vi "_SILAR 2016.vi"() -> ()   [LabVIEW 2016]
uses:
  <vilib>/LabVIEW Interface for Arduino/LabVIEW Interface for Arduino.lvlib
panel:
  in  "?":T1(tab)
  in  "Запись в файл":bool=TRUE
  in  "Необходимая температура":dbl[](array[numeric])=[90.0, 0.0, 0.0, 0.0]
  in  "Кол-во погружений в каждый стакан":i32[](array[numeric])=[1, 1, 1, 1]
  in  "Кол-во жидкости в каждом стакане [мл]":dbl[](array[numeric])=[70.0, 70.0, 70.0, 70.0]
  in  "Глубина погружения в раствор [мм]":dbl[](array[numeric])=[5.0, 5.0, 5.0, 5.0]
  in  "Опускания подложки до раствора":dbl[](array[numeric])=[2.9, 2.9, 2.9, 2.9]
  in  "Опускания подложки в растворе":dbl[](array[numeric])=[2.9, 2.9, 2.9, 2.9]
  in  "Подъема подложки из раствора":dbl[](array[numeric])=[2.9, 2.9, 2.9, 2.9]
  in  "Подъема подложки над раствором":dbl[](array[numeric])=[2.9, 2.9, 2.9, 2.9]
  in  "Нахождения в растворе":dbl[](array[numeric])=[1.0, 1.0, 1.0, 1.0] caption="Время нахождения в растворе (секунды)"
  in  "Задержки после подъема из раствора":dbl[](array[numeric])=[0.0, 0.0, 0.0, 0.0]
  in  "Оператор":string="Матюшкин"
  in  "Образец":string
  in  "COM порт":refnum<visa-resource-name>="COM6"
  in  "Кол-во циклов наслаивания":i32=1
  in  "Кол-во используемых растворов":i32(ring)=1 items=["Один"=1, "Два"=2, "Три"=3, "Четыре"=4]
  in  "Высота стакана [мм]":dbl=81.2
  in  "Высота подложки [мм]":dbl=22.0
  in  "Режим погружения подложки":u16(ring) items=["Частичный", "Полный"]
  in  "Запуск":bool
  in  "Выход из программы":bool
  in  "Включение нагрева":bool=TRUE
  in  "Считать данные":bool
  in  "Путь к файлу":path=path "C:/Users/user/Dropbox/SILAR/Devic"
  out "Время Темп":dbl=7.964
  out "Текущая темп. 3":dbl
  out "Нагрева":timestamp=timestamp(-14399.531 s since 1904-01-01) format="%<%H:%M:%S>T"
  out "До конца процесса":timestamp=timestamp(-14399.531 s since 1904-01-01) format="%<%H:%M:%S>T"
  out "С начала процесса":timestamp=timestamp(-14399.531 s since 1904-01-01) format="%<%H:%M:%S>T"
  out "Всего процесса":timestamp=timestamp(-14399.531 s since 1904-01-01) format="%<%H:%M:%S>T"
  out "Процесс выполнения":dbl(slide) scale=0.0..1.0
  out "Текущая темп. 1":dbl
  out "Текущая темп. 4":dbl
  out "Текущая темп. 2":dbl
  out "Текущий цикл":dbl
  out "Всего циклов":i32=2
  in  "Запуск процесса":bool
  out "Indic":bool[](array[boolean])
  out "2":bool
  out "1":bool
  out "3":bool
  out "Стакакан 1":dbl(slide) scale=0.0..81.0
  out "Термометр 1":dbl(slide) scale=20.0..90.0 scale format="%#_3g"
  out "Стакакан 2":dbl(slide) scale=0.0..81.0
  out "Термометр 2":dbl(slide) scale=20.0..90.0 scale format="%#_3g"
  out "Стакакан 3":dbl(slide) scale=0.0..81.0
  out "Термометр 3":dbl(slide) scale=20.0..90.0 scale format="%#_3g"
  out "Стакакан 4":dbl(slide) scale=0.0..81.0
  out "Термометр 4":dbl(slide) scale=20.0..90.0 scale format="%#_3g"
  out "Текущее кол-во погружений в каждый стакан":i32[](array[numeric])
  in  "Остановка":bool
  out "Нагрев завершен":bool
  out "Нагрев включен":bool
  # "Вкл"
  # "Выкл"
  # "Параметры на каждом стакане"
  # "1              2             3             4"
  # "Температура [градусы Цельсия]"
  # "Скорость [мм/с] (max 2,9 мм/с)"
  # "Время [c]"
  # "Параметры процесса"
  # "Вкл"
  # "Выкл"
  # "Считывание параметров процесса"
  # "Время"
  # "1"
  # "2"
  # "3"
  # "4"
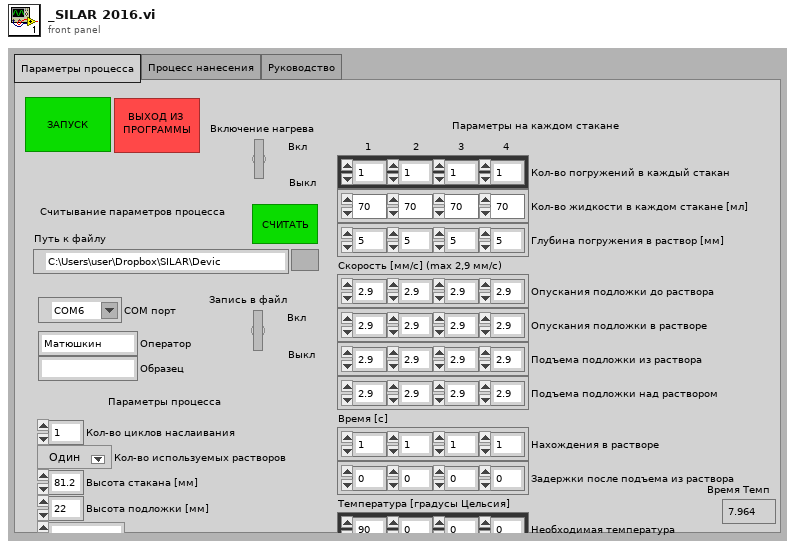
[diagram p1: front panel]
types:
  T1 = enum32{"Параметры процесса", "Процесс нанесения", "Руководство"}
  T2 = typedef "LabVIEW Interface for Arduino.lvlib/Arduino Resource.ctl" = cluster{"VISA resource":refnum<visa-resource-name>, "Board Type":T3, "Connection Type":enum8{"USB / Serial"}, "Bytes Per Packet (15)":u8}
  T3 = typedef "LabVIEW Interface for Arduino.lvlib/Board Type.ctl" = enum16{"Uno", "Dimuelanove w/Atmega 328", "Mega 2560"}
  T4 = enum32{"Параметры процесса", "Процесс нанесения"}
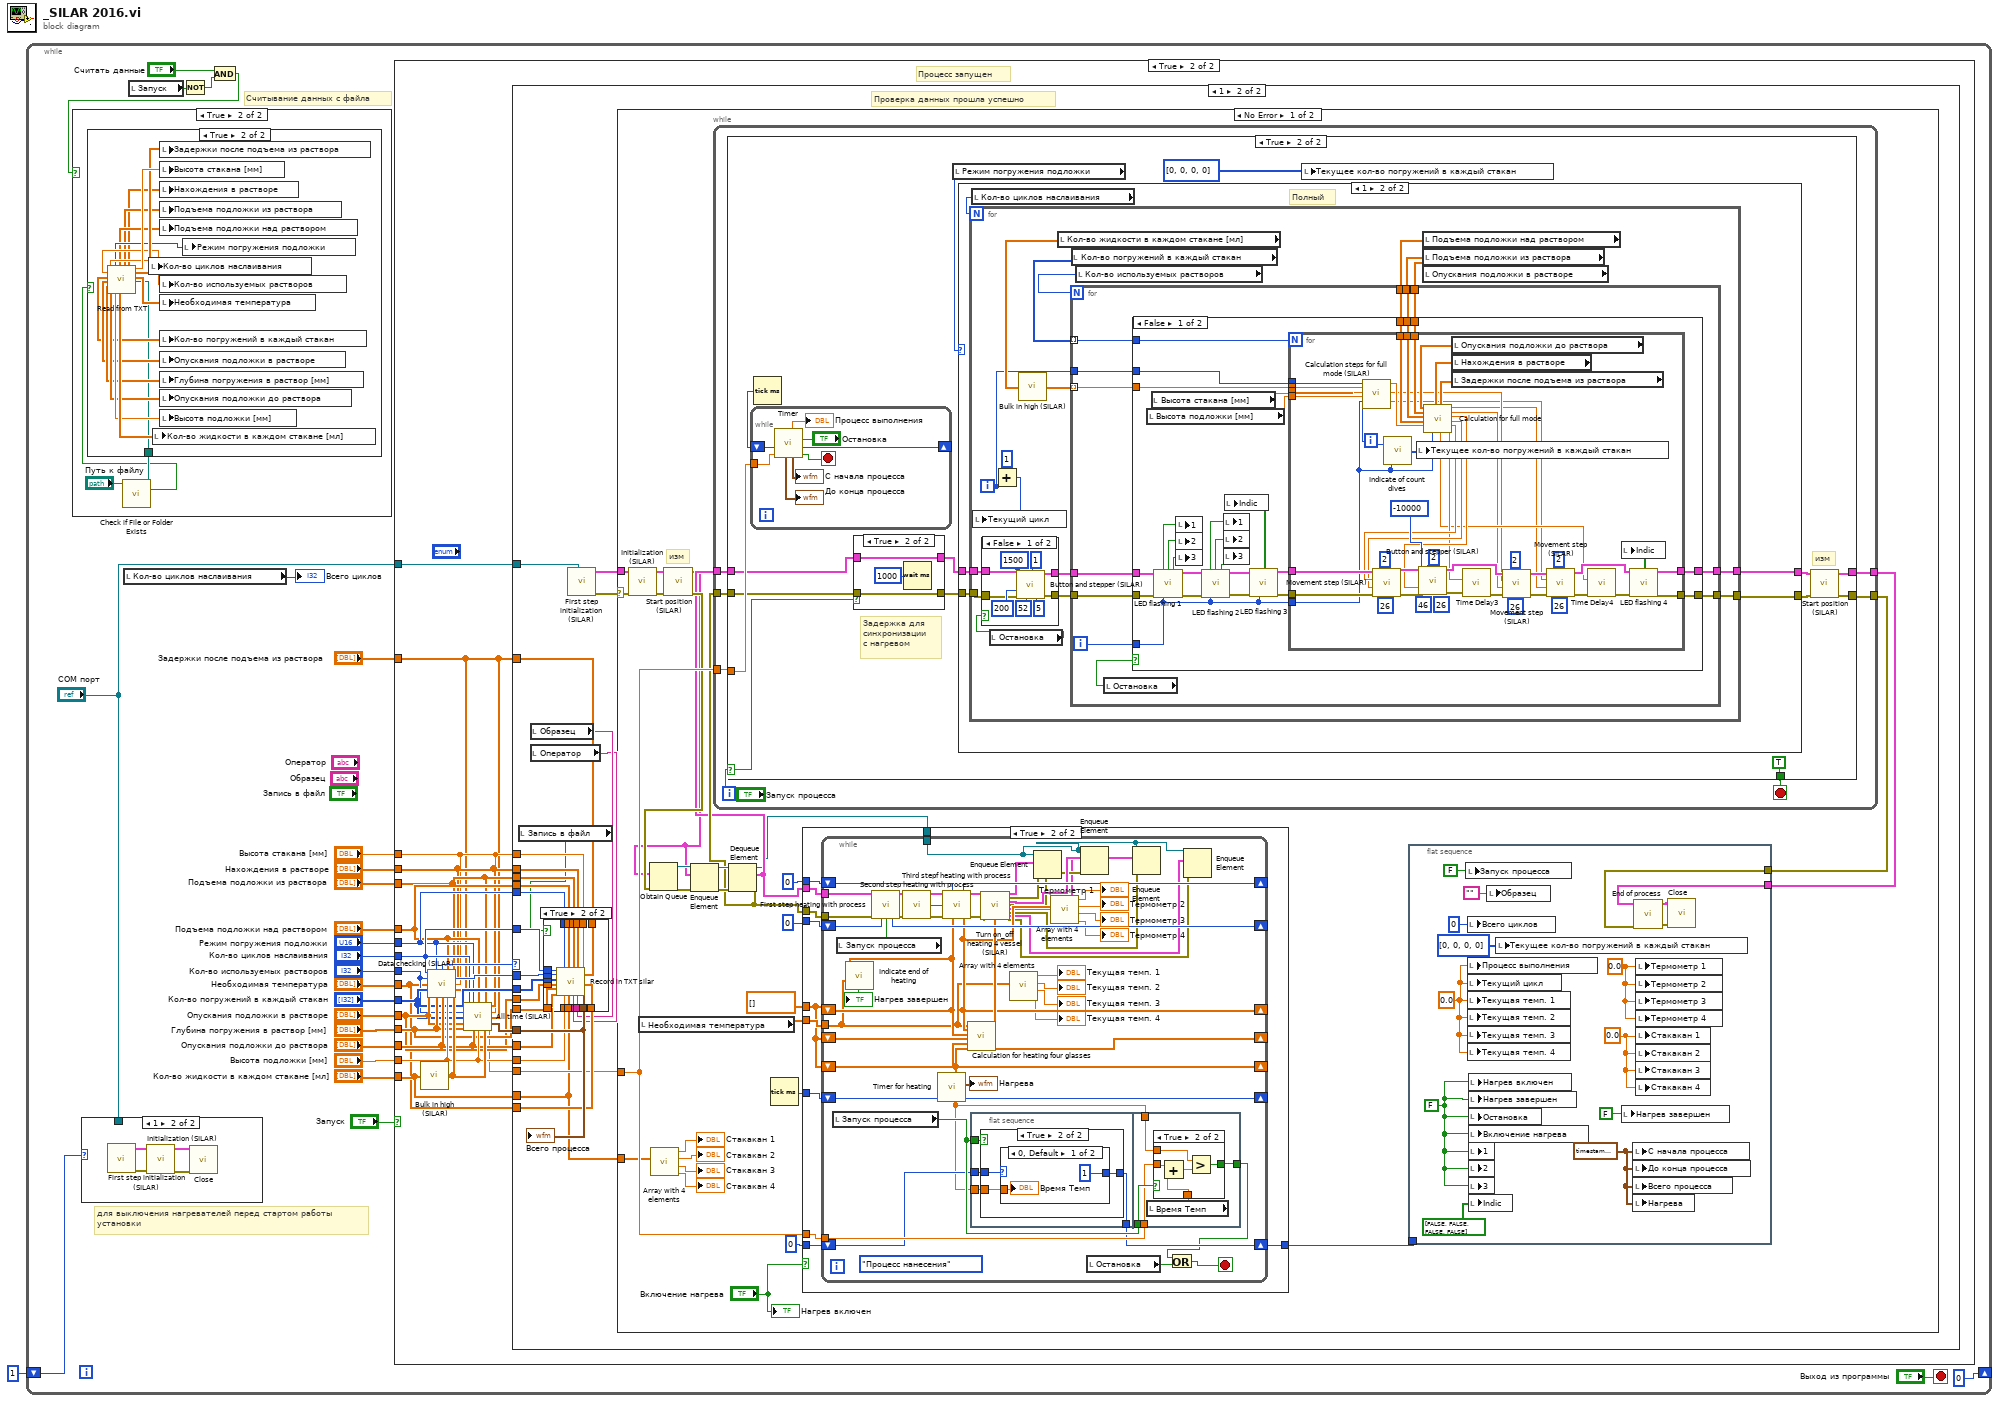
[diagram p0: block diagram]
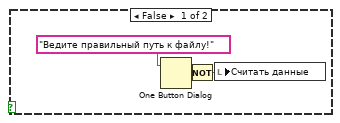
[diagram p4: hidden frame]
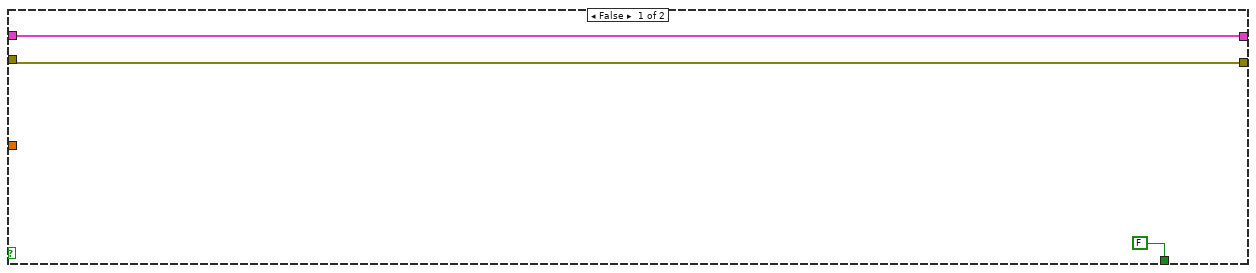
[diagram p8: hidden frame]
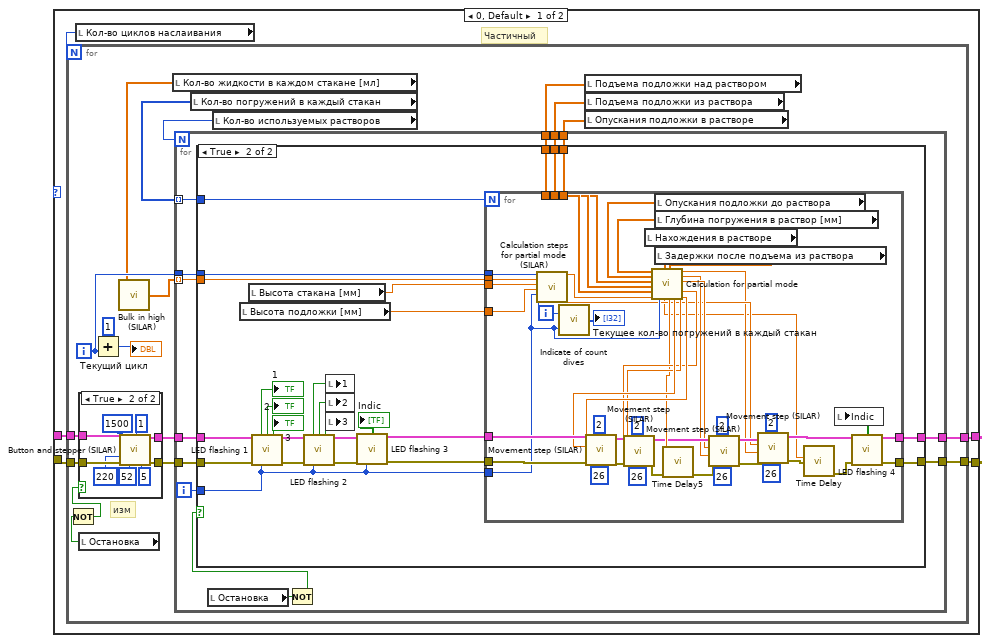
[diagram p10: hidden frame]
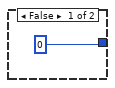
[diagram p15: hidden frame]
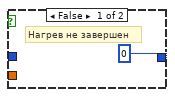
[diagram p16: hidden frame]
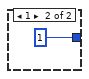
[diagram p17: hidden frame]
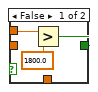
[diagram p18: hidden frame]
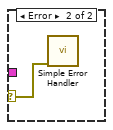
[diagram p19: hidden frame]
diagram:
  n1 = while {
    shift-right: [0 ("Всего циклов")] -> _
    shift-left: 1 -> [w3]
    stop <- "Выход из программы" stop-if-true
    # "для выключения нагревателей перед стартом работы\nустановки"
    # "Cчитывание данных с файла"
    n2 = case shown="1" w3 {
      tunnel: "COM порт" -> [_ _]
      frame 0, Default {
      }
      frame 1 {
        n3 = call "First step initialization (SILAR).vi"() -> ("Error Out"=w29:errorcluster, "Arduino Resource Out"=w30:T2)  [unwired: 10 in]
        n4 = call "Initialization (SILAR).vi"("Error In"=w29, "Arduino Resource In"=w30) -> ("Error Out"=w27:errorcluster, "Arduino Resource Out"=w28:T2)  [unwired: 8 in]
        n5 = call <vilib>:"Close.vi"("Arduino Resource"=w28, "error in"=w27) -> ()  [unwired: 13 in, 1 out]
      }
    }
    n6 = local read "Кол-во циклов наслаивания"() -> (→"Всего циклов":i32)
    n7 = local read "Запуск"() -> (w25:bool)
    n8 = Not(x=w25) -> (.not. x?=w22:bool)
    n9 = And(x="Считать данные", y=w22) -> (x .and. y?=w24:bool)
    n10 = case shown="True" w24 {
      frame False {
      }
      frame True {
        n11 = call <vilib>:"Check if File or Folder Exists.vi"("path"="Путь к файлу") -> ("file or folder exists?"=w31:bool, "dup path"=w32:path)  [unwired: 8 in, 1 out]
        n12 = case shown="True" w31 {
          tunnel: w32 -> [_ w37]
          frame False {
            n13 = One Button Dialog(message="Ведите правильный путь к файлу!") -> (true=w34:bool)  [unwired: 1 in]
            n14 = Not(x=w34) -> (.not. x?=w35:bool)
            n15 = local write "Считать данные"(w35) -> ()
          }
          frame True {
            n16 = call "Read from TXT.vi"("Файл с параметрами"=w37) -> ("Кол-во циклов наслаивания"=w42:dbl, "Кол-во используемых растворов"=w43:dbl, "Кол-во погружений в каждый раствор:"=w44:dbl[], "Опускания подложки в растворе:"=w45:dbl[], "Глубина погружения в раствор [мм]:"=w46:dbl[], "Опускания подложки до раствора:"=w47:dbl[], "Режим погружения"=w41:i32, "Высота подложки [мм]"=w48:dbl, "Подъем подложки над раствором:"=w40:dbl[], "Кол-во жидкости в стакане [мл]:"=w49:dbl[], "Подъема подложки из раствора:"=w39:dbl[], "Нахождения в растворе:"=w38:dbl[], "Высота стакана [мм]"=w52:dbl, "Задержки после подъема из раствора:"=w51:dbl[], "Температура в стаканах:"=w50:dbl[])  [unwired: 3 in, 1 out]
            n17 = local write "Кол-во циклов наслаивания"(w42) -> ()
            n18 = local write "Кол-во жидкости в каждом стакане [мл]"(w49) -> ()
            n19 = local write "Задержки после подъема из раствора"(w51) -> ()
            n20 = local write "Высота стакана [мм]"(w52) -> ()
            n21 = local write "Нахождения в растворе"(w38) -> ()
            n22 = local write "Подъема подложки из раствора"(w39) -> ()
            n23 = local write "Подъема подложки над раствором"(w40) -> ()
            n24 = local write "Кол-во используемых растворов"(w43) -> ()
            n25 = local write "Необходимая температура"(w50) -> ()
            n26 = local write "Кол-во погружений в каждый стакан"(w44) -> ()
            n27 = local write "Опускания подложки в растворе"(w45) -> ()
            n28 = local write "Глубина погружения в раствор [мм]"(w46) -> ()
            n29 = local write "Опускания подложки до раствора"(w47) -> ()
            n30 = local write "Высота подложки [мм]"(w48) -> ()
            n31 = local write "Режим погружения подложки"(w41) -> ()
          }
        }
      }
    }
    n32 = case shown="True" "Запуск" {
      tunnel: "Задержки после подъема из раствора" -> [_ w56]
      tunnel: "Высота стакана [мм]" -> [_ w57]
      tunnel: "Нахождения в растворе" -> [_ w58]
      tunnel: "Подъема подложки из раствора" -> [_ w59]
      tunnel: "Подъема подложки над раствором" -> [_ w60]
      tunnel: "Режим погружения подложки" -> [_ w61]
      tunnel: "Кол-во циклов наслаивания" -> [_ w62]
      tunnel: "Кол-во используемых растворов" -> [_ w63]
      tunnel: "Необходимая температура" -> [_ w55]
      tunnel: "Кол-во погружений в каждый стакан" -> [_ w64]
      tunnel: "Опускания подложки в растворе" -> [_ w65]
      tunnel: "Глубина погружения в раствор [мм]" -> [_ w66]
      tunnel: "Опускания подложки до раствора" -> [_ w67]
      tunnel: "Высота подложки [мм]" -> [_ w68]
      tunnel: "Кол-во жидкости в каждом стакане [мл]" -> [_ w69]
      tunnel: "COM порт" -> [_ w53]
      frame False {
      }
      frame True {
        # "Процесс запущен"
        n33 = call "Bulk in high (SILAR).vi"("Кол-во жидкости в каждом стакане (мл)"=w69) -> ("Кол-во жидкости в каждом стакане (мм)"=w72:dbl[])
        n34 = call "Data checking (SILAR).vi"("Необходимое кол-во циклов"=w62, "Режим погружения подложки"=w61, "Подъема подложки над раствором"=w60, "Подъема подложки из раствора"=w59, "Кол-во используемых растворов"=w63, "Время нахождения в растворе (секунды)"=w58, "Необходимая температура"=w55, "Высота стакана"=w57, "Кол-во погружений в каждый стакан за один цикл"=w64, "Задержки после подъема из раствора"=w56, "Опускания подложки в раствор"=w65, "Глубина погружения в раствор"=w66, "Опускания подложки до раствора"=w67, "Высота подложки"=w68, "Кол-во жидкости в каждом стакане (мм)"=w72) -> ("ПРОВЕРКА"=w71:i16)
        n35 = call "All time (SILAR).vi"("Необходимое кол-во циклов"=w62, "Режим погружения подложки"=w61, "Подъема подложки над раствором"=w60, "Подъема подложки из раствора"=w59, "Нахождения в растворе (секунды)"=w58, "Кол-во используемых растворов"=w63, "Высота стакана (мм)"=w57, "Кол-во погружений в каждый стакан за один цикл"=w64, "Задержка после подъема из раствора (секунды)"=w56, "Опускания подложки в раствор"=w65, "Глубина погружения в раствор (мм)"=w66, "Опускания подложки до раствора"=w67, "Высота подложки (мм)"=w68, "Кол-во жидкости в каждом стакане (мм)"=w72) -> (10:"Все время"=w70:timestamp, 15:"Все время"=w54:dbl)
        n36 = case shown="1" w71 {
          tunnel: w70 -> [_ w95]
          tunnel: w69 -> [_ w77]
          tunnel: w68 -> [_ w94]
          tunnel: w67 -> [_ w93]
          tunnel: w66 -> [_ w92]
          tunnel: w65 -> [_ w91]
          tunnel: w64 -> [_ w90]
          tunnel: w63 -> [_ w89]
          tunnel: w62 -> [_ w88]
          tunnel: w61 -> [_ w87]
          tunnel: w60 -> [_ w86]
          tunnel: w59 -> [_ w85]
          tunnel: w58 -> [_ w84]
          tunnel: w57 -> [_ w83]
          tunnel: w56 -> [_ w82]
          tunnel: w55 -> [_ w81]
          tunnel: w54 -> [_ w78]
          tunnel: w53 -> [_ w76]
          frame 0, Default {
          }
          frame 1 {
            # "Проверка данных прошла успешно"
            n37 = local read "Запись в файл"() -> (w75:bool)
            n38 = local read "Образец"() -> (w74:string)
            n39 = local read "Оператор"() -> (w73:string)
            n40 = case shown="True" w75 {
              tunnel: w73 -> [_ w113]
              tunnel: w74 -> [_ w112]
              tunnel: w95 -> [_ w111]
              tunnel: w94 -> [_ w110]
              tunnel: w93 -> [_ w109]
              tunnel: w92 -> [_ w108]
              tunnel: w91 -> [_ w107]
              tunnel: w90 -> [_ w106]
              tunnel: w89 -> [_ w105]
              tunnel: w88 -> [_ w104]
              tunnel: w87 -> [_ w103]
              tunnel: w86 -> [_ w102]
              tunnel: w85 -> [_ w101]
              tunnel: w84 -> [_ w100]
              tunnel: w83 -> [_ w99]
              tunnel: w82 -> [_ w98]
              tunnel: w81 -> [_ w97]
              tunnel: w77 -> [_ w96]
              frame False {
              }
              frame True {
                n41 = call "Record in TXT silar.vi"("Кол-во циклов"=w104, "Кол-во используемых растворов"=w105, "Кол-во погружений в каждый стакан"=w106, "Опускания подложки в растворе"=w107, "Глубина погружения в раствор [мм]"=w108, "Опускания подложки до раствора"=w109, "Режим погружения подложки"=w103, "Высота подложки [мм]"=w110, "Подъема подложки над раствором"=w102, "Кол-во жидкости в каждом стакане [мл]"=w96, "Подъема подложки из раствора"=w101, "Оператор"=w113, "Нахождения в растворе"=w100, "Получаемый образец"=w112, "Высота стакана [мм]"=w99, "Задержки после подъема из раствора"=w98, "Необходимая температура"=w97, "Все время процесса"=w111) -> ()  [unwired: 2 in]
              }
            }
            n42 = call "First step initialization (SILAR).vi"("COM порт"=w76) -> ("Error Out"=w80:errorcluster, "Arduino Resource Out"=w79:T2)  [unwired: 9 in]
            n43 = case shown="No Error" w80 {
              selector: w80 -> [w141 w524]
              tunnel: w79 -> [w142 _]
              tunnel: w78 -> [w132 _]
              tunnel: w77 -> [w131 _]
              frame No Error {
                # "изм"
                n44 = call "Initialization (SILAR).vi"("Error In"=w141, "Arduino Resource In"=w142) -> ("Error Out"=w139:errorcluster, "Arduino Resource Out"=w140:T2)  [unwired: 8 in]
                n45 = local read "Необходимая температура"() -> (w138:dbl[])
                n46 = call "Array with 4 elements.vi"("Array with 4 elements"=w131) -> ("element 3"=→"Стакакан 4":dbl, "element 2"=→"Стакакан 3":dbl, "element 1"=→"Стакакан 2":dbl, "element 0"=→"Стакакан 1":dbl)  [unwired: 7 in]
                n47 = call "Start position (SILAR).vi"("Error In"=w139, "Arduino Resource In"=w140) -> ("Error Out"=w119:errorcluster, "Arduino Resource Out"=w115:T2)  [unwired: 8 in]
                n48 = Obtain Queue(element data type=w115, error in (no error)=w119) -> (queue out=w123:refnum<queue>, error out=w120:errorcluster)  [unwired: 3 in, 1 out]
                n49 = Enqueue Element(queue=w123, element=w115, error in (no error)=w120) -> (queue out=w122:refnum<queue>, error out=w121:errorcluster)  [unwired: 1 in, 1 out]
                n50 = Dequeue Element(queue=w122, error in (no error)=w121) -> (queue out=w116:refnum<queue>, element=w117:T2, error out=w118:errorcluster)  [unwired: 1 in, 1 out]
                n51 = while {
                  tunnel: w132 -> [w164]
                  tunnel: [w163] -> w129
                  tunnel: [w162] -> w130
                  tunnel: w117 -> [w161]
                  tunnel: w118 -> [w160]
                  stop <- w159 stop-if-true
                  n52 = case shown="True" "Запуск процесса" {
                    selector: "Запуск процесса" -> [_ w172]
                    tunnel: w164 -> [_ w178]
                    tunnel: [w167 w168] -> w163
                    tunnel: [w166 w169] -> w162
                    tunnel: w161 -> [w167 w174]
                    tunnel: w160 -> [w166 w173]
                    tunnel: [FALSE TRUE] -> w159
                    frame False {
                    }
                    frame True {
                      # "изм"
                      # "Задержка для\nсинхронизации\nс нагревом"
                      n53 = Tick Count (ms)() -> (millisecond timer value=w179:u32)
                      n54 = while {
                        shift-right: [w193] -> _
                        shift-left: w179 -> [w194]
                        tunnel: w178 -> [w188]
                        stop <- w192 stop-if-true
                        n55 = call "Timer.vi"("Остановка процесса"="Остановка", "Рассчитанное время"=w188, "shift before"=w194) -> ("end time"=w192:bool, "shift after"=w193:u32, "Время с начала процесса"=→"С начала процесса":timestamp, "Процесс выполнения (шкала)"=→"Процесс выполнения":dbl, "Осталось времени \nдо конца процесса"=→"До конца процесса":timestamp)  [unwired: 4 in]
                      }
                      n56 = case shown="True" w172 {
                        tunnel: [w182 w186] -> w176
                        tunnel: w173 -> [w182 w186]
                        tunnel: w174 -> [w183 w185]
                        tunnel: [w183 w185] -> w175
                        frame False {
                        }
                        frame True {
                          n57 = Wait (ms)(milliseconds to wait=u32 1000) -> ()  [unwired: 1 out]
                        }
                      }
                      n58 = local read "Режим погружения подложки"() -> (w181:u16)
                      n59 = case shown="1" w181 {
                        tunnel: w175 -> [w199 w322]
                        tunnel: w176 -> [w198 w321]
                        tunnel: [w196 w319] -> w171
                        tunnel: [w195 w318] -> w170
                        frame 0, Default {
                          # "Частичный"
                          n60 = local read "Кол-во циклов наслаивания"() -> (w197:i32)
                          n61 = for {
                            N: w197 -> [_]
                            tunnel: w199 -> [w217]
                            tunnel: w198 -> [w216]
                            tunnel: [w203] -> w196
                            tunnel: [w202] -> w195
                            i -> [w209]
                            # "изм"
                            n62 = local read "Остановка"() -> (w200:bool)
                            n63 = Not(x=w200) -> (.not. x?=w201:bool)
                            n64 = case shown="True" w201 {
                              tunnel: w217 -> [w219 w224]
                              tunnel: w216 -> [w218 w223]
                              tunnel: [w218 w222] -> w212
                              tunnel: [w219 w221] -> w211
                              frame False {
                              }
                              frame True {
                                n65 = call "Button and stepper (SILAR).vi"("Arduino Resource In"=w224, "Шаговый двигатель №"=u8 1 ("Stepper #"), "Кол-во шагов"=i16 1500 ("# of Steps to Move"), "Скорость двигателя"=i16 220 ("Set Speed (Steps per Second)"), "Error In"=w223, "Контакт концевика"=u8 52 ("Digital I/O Pin (0)"), "ENABLE контакт"=u8 5 ("ENABLE Pin")) -> ("Arduino Resource Out"=w221:T2, "Error Out"=w222:errorcluster)  [unwired: 7 in]
                              }
                            }
                            n66 = Add(x=1, y=w209) -> (x+y=→"Текущий цикл":i32)
                            n67 = local read "Кол-во жидкости в каждом стакане [мл]"() -> (w208:dbl[])
                            n68 = call "Bulk in high (SILAR).vi"("Кол-во жидкости в каждом стакане (мл)"=w208) -> ("Кол-во жидкости в каждом стакане (мм)"=w207:dbl[])
                            n69 = local read "Кол-во погружений в каждый стакан"() -> (w210:i32[])
                            n70 = local read "Кол-во используемых растворов"() -> (w213:i32)
                            n71 = local read "Подъема подложки над раствором"() -> (w206:dbl[])
                            n72 = local read "Подъема подложки из раствора"() -> (w205:dbl[])
                            n73 = local read "Опускания подложки в растворе"() -> (w204:dbl[])
                            n74 = for {
                              N: w213 -> [_]
                              tunnel: w212 -> [w241]
                              tunnel: w211 -> [w240]
                              tunnel: w210 -> [w239] mode=indexing
                              tunnel: w209 -> [w238]
                              tunnel: w207 -> [w237] mode=indexing
                              tunnel: w206 -> [w236]
                              tunnel: w205 -> [w235]
                              tunnel: w204 -> [w234]
                              tunnel: [w233] -> w203
                              tunnel: [w232] -> w202
                              i -> [w229]
                              n75 = local read "Остановка"() -> (w231:bool)
                              n76 = Not(x=w231) -> (.not. x?=w230:bool)
                              n77 = case shown="True" w230 {
                                tunnel: w241 -> [w242 w269]
                                tunnel: w240 -> [w243 w268]
                                tunnel: w239 -> [_ w267]
                                tunnel: w238 -> [_ w266]
                                tunnel: w237 -> [_ w265]
                                tunnel: w236 -> [_ w260]
                                tunnel: w235 -> [_ w259]
                                tunnel: w234 -> [_ w258]
                                tunnel: [w243 w257] -> w233
                                tunnel: [w242 w256] -> w232
                                tunnel: w229 -> [_ w255]
                                frame False {
                                }
                                frame True {
                                n78 = local read "Высота подложки [мм]"() -> (w263:dbl)
                                n79 = local read "Высота стакана [мм]"() -> (w264:dbl)
                                n80 = call "LED flashing 1.vi"("Arduino Resource In"=w268, "Error Out In"=w269, "Текущий раствор"=w255) -> ("1"=→"1":bool, "2"=→"2":bool, "3"=→"3":bool, "Arduino Resource Out"=w251:T2, "Error Out"=w250:errorcluster)  [unwired: 8 in]
                                n81 = call "LED flashing 2.vi"("Arduino Resource In"=w251, "Error In"=w250, "Текущий раствор"=w255) -> ("1"=w247:bool, "2"=w248:bool, "3"=w249:bool, "Arduino Resource Out"=w246:T2, "Error Out"=w245:errorcluster)  [unwired: 8 in]
                                n82 = local write "1"(w247) -> ()
                                n83 = local write "2"(w248) -> ()
                                n84 = local write "3"(w249) -> ()
                                n85 = call "LED flashing 3.vi"("Arduino Resource In"=w246, "Error In"=w245, "Текущий раствор"=w255) -> ("1           2           3          4"=→"Indic":bool[], "Arduino Resource Out"=w262:T2, "Error Out"=w261:errorcluster)  [unwired: 10 in]
                                n86 = for {
                                N: w267 -> [_]
                                tunnel: w266 -> [w317]
                                tunnel: w265 -> [w316]
                                tunnel: w264 -> [w315]
                                tunnel: w263 -> [w314]
                                tunnel: w255 -> [w309]
                                tunnel: w262 -> [w311]
                                tunnel: w261 -> [w310]
                                tunnel: w260 -> [w307]
                                tunnel: w259 -> [w306]
                                tunnel: w258 -> [w305]
                                tunnel: [w299] -> w257
                                tunnel: [w298] -> w256
                                i -> [w312]
                                n87 = call "Calculation steps for partial mode (SILAR).vi"("Loop iteration для кол-ва циклов"=w317, "Кол-во жидкости в каждом стакане [мм]"=w316, "Высота стакана [мм]"=w315, "Высота подложки [мм]"=w314, "Loop iteration для кол-ва используемых растворов"=w309, "Loop iteration для кол-ва погружений в каждый стакан"=w312) -> ("Кол-во шагов до раствора"=w308:dbl, "Кол-во шагов над раствором"=w283:dbl)  [unwired: 12 in]
                                n88 = call "Indicate of count dives.vi"("Текущий раствор"=w309, "Текущее погружение"=w312) -> ("Текущее кол-во погружений в каждый стакан"=→"Текущее кол-во погружений в каждый стакан":i32[])
                                n89 = local read "Нахождения в растворе"() -> (w302:dbl[])
                                n90 = local read "Опускания подложки до раствора"() -> (w304:dbl[])
                                n91 = local read "Глубина погружения в раствор [мм]"() -> (w303:dbl[])
                                n92 = local read "Задержки после подъема из раствора"() -> (w301:dbl[])
                                n93 = call "Calculation for partial mode.vi"("Глубина погружения в раствор [мм]"=w303, "Опускания подложки до раствора"=w304, "Опускания подложки в растворе"=w305, "Подъема подложки из раствора"=w306, "Подъема подложки над раствором"=w307, "Steps for partial mode"=w308, "Текущий раствор"=w309, "Нахождения в растворе"=w302, "Задержки после подъема из раствора"=w301) -> ("Время задержки после подъема"=w279:dbl, "Время нахождения в растворе"=w290:dbl, "Кол-во шагов 1"=w297:dbl, "Скорость 4"=w282:dbl, "Скорость 3"=w286:dbl, "Кол-во шагов 3"=w287:dbl, "Скорость 2"=w293:dbl, "Кол-во шагов 2"=w292:dbl, "Скорость 1"=w296:dbl)  [unwired: 2 in]
                                n94 = call "Movement step (SILAR).vi"("ENABLE контакт"=u8 26 ("ENABLE Pin"), "Шаговый двигатель №"=u8 2 ("Stepper #"), "Error In"=w310, "Скорость"=w296, "Кол-во шагов"=w297, "Arduino Resource In"=w311) -> ("Error Out"=w294:errorcluster, "Arduino Resource Out"=w295:T2)  [unwired: 4 in]
                                n95 = call "Movement step (SILAR).vi"("ENABLE контакт"=u8 26 ("ENABLE Pin"), "Шаговый двигатель №"=u8 2 ("Stepper #"), "Error In"=w294, "Скорость"=w293, "Кол-во шагов"=w292, "Arduino Resource In"=w295) -> ("Error Out"=w291:errorcluster, "Arduino Resource Out"=w289:T2)  [unwired: 4 in]
                                n96 = call "Time Delay5"("error in (no error)"=w291, "Delay Time (s)"=w290) -> ("error out"=w288:errorcluster)  [unwired: 9 in]
                                n97 = call "Movement step (SILAR).vi"("ENABLE контакт"=u8 26 ("ENABLE Pin"), "Шаговый двигатель №"=u8 2 ("Stepper #"), "Error In"=w288, "Скорость"=w286, "Кол-во шагов"=w287, "Arduino Resource In"=w289) -> ("Error Out"=w284:errorcluster, "Arduino Resource Out"=w285:T2)  [unwired: 4 in]
                                n98 = call "Movement step (SILAR).vi"("ENABLE контакт"=u8 26 ("ENABLE Pin"), "Шаговый двигатель №"=u8 2 ("Stepper #"), "Error In"=w284, "Скорость"=w282, "Кол-во шагов"=w283, "Arduino Resource In"=w285) -> ("Error Out"=w280:errorcluster, "Arduino Resource Out"=w281:T2)  [unwired: 4 in]
                                n99 = call "Time Delay"("error in (no error)"=w280, "Delay Time (s)"=w279) -> ("error out"=w270:errorcluster)  [unwired: 9 in]
                                n100 = call "LED flashing 4.vi"("Arduino Resource In"=w281, "Error In"=w270) -> ("1           2           3          4"=w300:bool[], "Arduino Resource Out"=w299:T2, "Error Out"=w298:errorcluster)  [unwired: 11 in]
                                n101 = local write "Indic"(w300) -> ()
                                }
                                }
                              }
                            }
                          }
                        }
                        frame 1 {
                          # "Полный"
                          n102 = local read "Кол-во циклов наслаивания"() -> (w320:i32)
                          n103 = for {
                            N: w320 -> [_]
                            tunnel: w322 -> [w338]
                            tunnel: w321 -> [w337]
                            tunnel: [w328] -> w319
                            tunnel: [w327] -> w318
                            i -> [w330]
                            n104 = local read "Остановка"() -> (w323:bool)
                            n105 = case shown="False" w323 {
                              tunnel: w338 -> [w343 w350]
                              tunnel: w337 -> [w342 w349]
                              tunnel: [w341 w350] -> w333
                              tunnel: [w340 w349] -> w332
                              frame False {
                                n106 = call "Button and stepper (SILAR).vi"("Arduino Resource In"=w343, "Шаговый двигатель №"=u8 1 ("Stepper #"), "Кол-во шагов"=i16 1500 ("# of Steps to Move"), "Скорость двигателя"=i16 200 ("Set Speed (Steps per Second)"), "Error In"=w342, "Контакт концевика"=u8 52 ("Digital I/O Pin (0)"), "ENABLE контакт"=u8 5 ("ENABLE Pin")) -> ("Arduino Resource Out"=w341:T2, "Error Out"=w340:errorcluster)  [unwired: 7 in]
                              }
                              frame True {
                              }
                            }
                            n107 = Add(x=1, y=w330) -> (x+y=w329:i32)
                            n108 = local write "Текущий цикл"(w329) -> ()
                            n109 = local read "Кол-во жидкости в каждом стакане [мл]"() -> (w334:dbl[])
                            n110 = call "Bulk in high (SILAR).vi"("Кол-во жидкости в каждом стакане (мл)"=w334) -> ("Кол-во жидкости в каждом стакане (мм)"=w331:dbl[])
                            n111 = local read "Кол-во погружений в каждый стакан"() -> (w335:i32[])
                            n112 = local read "Кол-во используемых растворов"() -> (w336:i32)
                            n113 = local read "Подъема подложки над раствором"() -> (w326:dbl[])
                            n114 = local read "Подъема подложки из раствора"() -> (w325:dbl[])
                            n115 = local read "Опускания подложки в растворе"() -> (w324:dbl[])
                            n116 = for {
                              N: w336 -> [_]
                              tunnel: w335 -> [w360] mode=indexing
                              tunnel: w333 -> [w362]
                              tunnel: w332 -> [w361]
                              tunnel: w331 -> [w358] mode=indexing
                              tunnel: w330 -> [w359]
                              tunnel: [w357] -> w328
                              tunnel: [w356] -> w327
                              tunnel: w326 -> [w355]
                              tunnel: w325 -> [w354]
                              tunnel: w324 -> [w353]
                              i -> [w352]
                              n117 = local read "Остановка"() -> (w351:bool)
                              n118 = case shown="False" w351 {
                                tunnel: w362 -> [w388 w436]
                                tunnel: w361 -> [w387 w435]
                                tunnel: w360 -> [w375 _]
                                tunnel: w359 -> [w374 _]
                                tunnel: w358 -> [w373 _]
                                tunnel: [w368 w436] -> w357
                                tunnel: [w367 w435] -> w356
                                tunnel: w355 -> [w366 _]
                                tunnel: w354 -> [w365 _]
                                tunnel: w353 -> [w364 _]
                                tunnel: w352 -> [w363 _]
                                frame False {
                                n119 = local read "Высота подложки [мм]"() -> (w371:dbl)
                                n120 = local read "Высота стакана [мм]"() -> (w372:dbl)
                                n121 = call "LED flashing 1.vi"("Arduino Resource In"=w388, "Error Out In"=w387, "Текущий раствор"=w363) -> ("1"=w382:bool, "2"=w381:bool, "3"=w380:bool, "Arduino Resource Out"=w386:T2, "Error Out"=w383:errorcluster)  [unwired: 8 in]
                                n122 = local write "1"(w382) -> ()
                                n123 = local write "2"(w381) -> ()
                                n124 = local write "3"(w380) -> ()
                                n125 = call "LED flashing 2.vi"("Arduino Resource In"=w386, "Error In"=w383, "Текущий раствор"=w363) -> ("1"=w379:bool, "2"=w378:bool, "3"=w377:bool, "Arduino Resource Out"=w385:T2, "Error Out"=w384:errorcluster)  [unwired: 8 in]
                                n126 = local write "1"(w379) -> ()
                                n127 = local write "2"(w378) -> ()
                                n128 = local write "3"(w377) -> ()
                                n129 = call "LED flashing 3.vi"("Arduino Resource In"=w385, "Error In"=w384, "Текущий раствор"=w363) -> ("1           2           3          4"=w376:bool[], "Arduino Resource Out"=w370:T2, "Error Out"=w369:errorcluster)  [unwired: 10 in]
                                n130 = local write "Indic"(w376) -> ()
                                n131 = for {
                                N: w375 -> [_]
                                tunnel: w374 -> [w434]
                                tunnel: w373 -> [w433]
                                tunnel: w372 -> [w432]
                                tunnel: w371 -> [w431]
                                tunnel: w363 -> [w400]
                                tunnel: w370 -> [w416]
                                tunnel: w369 -> [w415]
                                tunnel: [w414] -> w368
                                tunnel: [w413] -> w367
                                tunnel: w366 -> [w406]
                                tunnel: w365 -> [w405]
                                tunnel: w364 -> [w404]
                                i -> [w430]
                                (unwired) u8 26 ("ENABLE Pin")
                                (unwired) u8 46 ("Digital I/O Pin (0)")
                                n132 = call "Calculation steps for full mode (SILAR).vi"("Loop iteration для кол-ва циклов"=w434, "Кол-во жидкости в каждом стакане [мм]"=w433, "Высота стакана [мм]"=w432, "Высота подложки [мм]"=w431, "Loop iteration для кол-ва используемых растворов"=w400, "Loop iteration для кол-ва погружений в каждый стакан"=w430) -> ("Кол-во шагов до раствора"=w399:dbl, "Кол-во шагов из раствора"=w393:dbl, "Кол-во шагов над раствором"=w391:dbl)  [unwired: 11 in]
                                n133 = call "Indicate of count dives.vi"("Текущий раствор"=w400, "Текущее погружение"=w430) -> ("Текущее кол-во погружений в каждый стакан"=w429:i32[])
                                n134 = local write "Текущее кол-во погружений в каждый стакан"(w429) -> ()
                                n135 = local read "Опускания подложки до раствора"() -> (w403:dbl[])
                                n136 = local read "Нахождения в растворе"() -> (w402:dbl[])
                                n137 = local read "Задержки после подъема из раствора"() -> (w401:dbl[])
                                n138 = call "Calculation for full mode.vi"("Опускания подложки до раствора"=w403, "Опускания подложки в растворе"=w404, "Подъема подложки из раствора"=w405, "Подъема подложки над раствором"=w406, "Steps for full mode"=w399, "Текущий раствор"=w400, "Нахождения в растворе"=w402, "Задержки после подъема из раствора"=w401) -> ("Время задержки после подъема"=w394:dbl, "Время нахождения в растворе"=w395:dbl, "Скорость 4"=w390:dbl, "Скорость 3"=w392:dbl, "Скорость 2"=w396:dbl, "Скорость 1"=w397:dbl, "Кол-во шагов 1"=w398:dbl)  [unwired: 5 in]
                                n139 = call "Movement step (SILAR).vi"("ENABLE контакт"=u8 26 ("ENABLE Pin"), "Шаговый двигатель №"=u8 2 ("Stepper #"), "Error In"=w415, "Скорость"=w397, "Кол-во шагов"=w398, "Arduino Resource In"=w416) -> ("Error Out"=w408:errorcluster, "Arduino Resource Out"=w409:T2)  [unwired: 4 in]
                                n140 = call "Button and stepper (SILAR).vi"("Arduino Resource In"=w409, "Шаговый двигатель №"=u8 2 ("Stepper #"), "Кол-во шагов"=i16 -10000 ("# of Steps to Move"), "Скорость двигателя"=w396, "Error In"=w408) -> ("Arduino Resource Out"=w411:T2, "Error Out"=w410:errorcluster)  [unwired: 9 in]
                                n141 = call "Time Delay3"("error in (no error)"=w410, "Delay Time (s)"=w395) -> ("error out"=w425:errorcluster)  [unwired: 9 in]
                                n142 = call "Movement step (SILAR).vi"("ENABLE контакт"=u8 26 ("ENABLE Pin"), "Шаговый двигатель №"=u8 2 ("Stepper #"), "Error In"=w425, "Скорость"=w392, "Кол-во шагов"=w393, "Arduino Resource In"=w411) -> ("Error Out"=w424:errorcluster, "Arduino Resource Out"=w423:T2)  [unwired: 4 in]
                                n143 = call "Movement step (SILAR).vi"("ENABLE контакт"=u8 26 ("ENABLE Pin"), "Шаговый двигатель №"=u8 2 ("Stepper #"), "Error In"=w424, "Скорость"=w390, "Кол-во шагов"=w391, "Arduino Resource In"=w423) -> ("Error Out"=w426:errorcluster, "Arduino Resource Out"=w427:T2)  [unwired: 4 in]
                                n144 = call "Time Delay4"("error in (no error)"=w426, "Delay Time (s)"=w394) -> ("error out"=w428:errorcluster)  [unwired: 9 in]
                                n145 = call "LED flashing 4.vi"("Arduino Resource In"=w427, "Error In"=w428) -> ("1           2           3          4"=w389:bool[], "Arduino Resource Out"=w414:T2, "Error Out"=w413:errorcluster)  [unwired: 11 in]
                                n146 = local write "Indic"(w389) -> ()
                                }
                                }
                                frame True {
                                }
                              }
                            }
                          }
                        }
                      }
                      n147 = local write "Текущее кол-во погружений в каждый стакан"(i32[] [0, 0, 0, 0] ("Текущее кол-во погружений в каждый стакан")) -> ()
                      n148 = call "Start position (SILAR).vi"("Error In"=w170, "Arduino Resource In"=w171) -> ("Error Out"=w169:errorcluster, "Arduino Resource Out"=w168:T2)  [unwired: 8 in]
                    }
                  }
                }
                n149 = Tick Count (ms)() -> (millisecond timer value=w134:u32)
                n150 = case shown="True" "Включение нагрева" {
                  tunnel: w117 -> [_ w448]
                  tunnel: w118 -> [_ w447]
                  tunnel: w138 -> [_ w444]
                  tunnel: dbl[] [] -> [_ w443]
                  tunnel: 0 -> [_ w446]
                  tunnel: 0 -> [_ w445]
                  tunnel: w134 -> [_ w442]
                  tunnel: 0 -> [_ w441]
                  tunnel: w132 -> [_ w440]
                  tunnel: w116 -> [_ w439]
                  tunnel: [0 w438] -> w114
                  frame False {
                  }
                  frame True {
                    n151 = while {
                      tunnel: w448 -> [w499]
                      tunnel: w447 -> [w495]
                      shift-right: [w470] -> _
                      shift-left: w443 -> [w477]
                      shift-right: [w484] -> _
                      shift-left: w443 -> [w483]
                      shift-right: [w497] -> _
                      shift-left: w446 -> [w498]
                      shift-right: [w488] -> _
                      shift-left: w445 -> [w489]
                      tunnel: w444 -> [w465]
                      shift-right: [w476] -> _
                      shift-left: w443 -> [w482]
                      shift-right: [w480] -> _
                      shift-left: w442 -> [w481]
                      shift-right: [w472] -> w438
                      shift-left: w441 -> [w473]
                      tunnel: w440 -> [w474]
                      tunnel: w439 -> [w452]
                      stop <- w449 stop-if-true
                      (unwired) T4."Процесс нанесения"
                      n152 = local read "Запуск процесса"() -> (w475:bool)
                      n153 = local read "Запуск процесса"() -> (w496:bool)
                      n154 = call "Indicate end of heating.vi"("Заданная температура"=w465, "Прошлая температура"=w477) -> ("Нагрев завершен"=→"Нагрев завершен":bool)  [unwired: 9 in]
                      n155 = call "First step heating with process.vi"("Arduino Resource In"=w499, "Error In"=w495, "shift left"=w498, "Запуск процесса"=w496) -> ("Arduino Resource Out"=w494:T2, "Shift right"=w497:i32, "Error Out"=w493:errorcluster)  [unwired: 9 in]
                      n156 = call "Second step heating with process.vi"("Arduino Resource In"=w494, "Error In"=w493) -> ("Arduino Resource Out"=w492:T2, "isWork"=w491:bool, "Error Out"=w490:errorcluster)  [unwired: 11 in]
                      n157 = call "Timer for heating.vi"("shift before"=w481) -> ("shift after"=w480:u32, "Время нагрева"=→"Нагрева":timestamp, "Текущее время"=w471:dbl, "Текущее время (array)"=w476:dbl[])  [unwired: 7 in]
                      n158 = call "Third stepf heating with process.vi"("Arduino Resource In"=w492, "Shift left"=w489, "Boolean from second step"=w491, "Error In"=w490, "Температура после shift register"=w477) -> ("Shift right"=w488:i32, "Arduino Resource Out"=w487:T2, "Текущая температура"=w470:dbl[], "Error Out"=w486:errorcluster)  [unwired: 7 in]
                      n159 = call "Calculation for heating four glasses.vi"("Заданная температура"=w465, "Текущая температура"=w470, "Прошлая температура"=w477, "Суммарная (прошлая) температура"=w483, "Время прошлое"=w482, "Время настоящее"=w476) -> ("Время во включенном состоянии"=w485:dbl[], "Суммарная температура"=w484:dbl[])  [unwired: 12 in]
                      n160 = flat-sequence {
                        tunnel: w475 -> [w503]
                        tunnel: w473 -> [w502]
                        tunnel: [w501] -> w472
                        tunnel: w471 -> [w500]
                        tunnel: w475 -> [w515]
                        tunnel: w471 -> [w514]
                        tunnel: w474 -> [w513]
                        tunnel: [w511] -> w450
                        frame #0 {
                          n161 = case shown="True" w503 {
                            tunnel: w502 -> [_ w507]
                            tunnel: w500 -> [_ w506]
                            tunnel: [0 w505] -> w501
                            frame False {
                              # "Нагрев не завершен"
                            }
                            frame True {
                              n162 = case shown="0, Default" w507 {
                                tunnel: w506 -> [w508 _]
                                tunnel: [1 1] -> w505
                                frame 0, Default {
                                "Время Темп" <- w508
                                }
                                frame 1 {
                                }
                              }
                            }
                          }
                        }
                        frame #1 {
                          n163 = local read "Время Темп"() -> (w512:dbl)
                          n164 = case shown="True" w515 {
                            tunnel: w513 -> [_ w521]
                            tunnel: [w517 w523] -> w511
                            tunnel: w514 -> [w516 w520]
                            tunnel: w512 -> [_ w519]
                            frame False {
                              n165 = Greater?(x=w516, y=1800.0) -> (0:w517:bool)
                            }
                            frame True {
                              n166 = Add(x=w521, y=w519) -> (x+y=w522:dbl)
                              n167 = Greater?(x=w520, y=w522) -> (0:w523:bool)
                            }
                          }
                        }
                      }
                      n168 = call "Turn on_off heating 4 vessel (SILAR).vi"("Arduino Resource In 1"=w487, "Error In 1"=w486, "t1 - время во включенном состоянии"=w485) -> ("Arduino Resource Out 1"=w460:T2, "error out 1"=w459:errorcluster, "Arduino Resource Out 2"=w458:T2, "error out 2"=w457:errorcluster, "Arduino Resource Out 3"=w455:T2, "error out 3"=w456:errorcluster, "Arduino Resource Out 4"=w454:T2, "error out 4"=w453:errorcluster)  [unwired: 17 in]
                      n169 = call "Array with 4 elements.vi"("Array with 4 elements"=w465) -> ("element 3"=→"Текущая темп. 4":dbl, "element 2"=→"Текущая темп. 3":dbl, "element 1"=→"Текущая темп. 2":dbl, "element 0"=→"Текущая темп. 1":dbl)  [unwired: 7 in]
                      n170 = Enqueue Element(queue=w452, element=w460, error in (no error)=w459) -> ()  [unwired: 1 in, 3 out]
                      n171 = call "Array with 4 elements.vi"("Array with 4 elements"=w470) -> ("element 3"=→"Термометр 4":dbl, "element 2"=→"Термометр 3":dbl, "element 1"=→"Термометр 2":dbl, "element 0"=→"Термометр 1":dbl)  [unwired: 7 in]
                      n172 = Enqueue Element(queue=w452, element=w458, error in (no error)=w457) -> ()  [unwired: 1 in, 3 out]
                      n173 = local read "Остановка"() -> (w451:bool)
                      n174 = Enqueue Element(queue=w452, element=w455, error in (no error)=w456) -> ()  [unwired: 1 in, 3 out]
                      n175 = Or(x=w450, y=w451) -> (x .or. y?=w449:bool)
                      n176 = Enqueue Element(queue=w452, element=w454, error in (no error)=w453) -> ()  [unwired: 1 in, 3 out]
                    }
                  }
                }
                n177 = flat-sequence {
                  tunnel: w130 -> [w155]
                  tunnel: w129 -> [w154]
                  tunnel: w114 -> [_]
                  frame #0 {
                    w148 = 0.0 ("Текущая темп. 1")
                    w149 = 0.0 ("Стакакан 1")
                    w150 = 0.0 ("Термометр 1")
                    w151 = timestamp(-14399.531 s since 1904-01-01) ("С начала процесса")
                    w153 = FALSE ("Остановка")
                    n178 = local write "Запуск процесса"(FALSE ("Запуск процесса")) -> ()
                    n179 = local write "Всего циклов"(0 ("Всего циклов")) -> ()
                    n180 = local write "Процесс выполнения"(w148) -> ()
                    n181 = local write "Текущий цикл"(w148) -> ()
                    n182 = local write "Текущая темп. 1"(w148) -> ()
                    n183 = local write "Текущая темп. 2"(w148) -> ()
                    n184 = local write "Текущая темп. 3"(w148) -> ()
                    n185 = local write "Текущая темп. 4"(w148) -> ()
                    n186 = local write "Нагрев включен"(w153) -> ()
                    n187 = local write "Нагрев завершен"(w153) -> ()
                    n188 = local write "Остановка"(w153) -> ()
                    n189 = local write "Включение нагрева"(w153) -> ()
                    n190 = local write "1"(w153) -> ()
                    n191 = local write "2"(w153) -> ()
                    n192 = local write "3"(w153) -> ()
                    n193 = local write "Indic"(bool[] [FALSE, FALSE, FALSE, FALSE] ("Indic")) -> ()
                    n194 = local write "Образец"("") -> ()
                    n195 = local write "Текущее кол-во погружений в каждый стакан"(i32[] [0, 0, 0, 0] ("Текущее кол-во погружений в каждый стакан")) -> ()
                    n196 = local write "Нагрев завершен"(FALSE ("Нагрев завершен")) -> ()
                    n197 = local write "С начала процесса"(w151) -> ()
                    n198 = local write "До конца процесса"(w151) -> ()
                    n199 = local write "Всего процесса"(w151) -> ()
                    n200 = local write "Нагрева"(w151) -> ()
                    n201 = call "End of process.vi"("Arduino Resource In"=w154, "Error In"=w155) -> ("Arduino Resource Out"=w157:T2, "Error Out"=w156:errorcluster)  [unwired: 16 in]
                    n202 = local write "Термометр 1"(w150) -> ()
                    n203 = local write "Термометр 2"(w150) -> ()
                    n204 = local write "Термометр 3"(w150) -> ()
                    n205 = local write "Термометр 4"(w150) -> ()
                    n206 = local write "Стакакан 1"(w149) -> ()
                    n207 = local write "Стакакан 2"(w149) -> ()
                    n208 = local write "Стакакан 3"(w149) -> ()
                    n209 = local write "Стакакан 4"(w149) -> ()
                    n210 = call <vilib>:"Close.vi"("Arduino Resource"=w157, "error in"=w156) -> ()  [unwired: 13 in, 1 out]
                  }
                }
                "Нагрев включен" <- "Включение нагрева"
              }
              frame Error {
                n211 = call <vilib>:"Simple Error Handler.vi"("error in (no error)"=w524) -> ()  [unwired: 4 in, 5 out]
              }
            }
            "Всего процесса" <- w95
          }
        }
      }
    }
  }
